vi "move X Relative.vi"(9 "Settings":T1, 10 "Speed X":i32, 11 "x mm":dbl) -> ()   [LabVIEW 2017]
uses:
  Settings/Settings-Control.ctl
  ICNC/ICNC2.lvlib
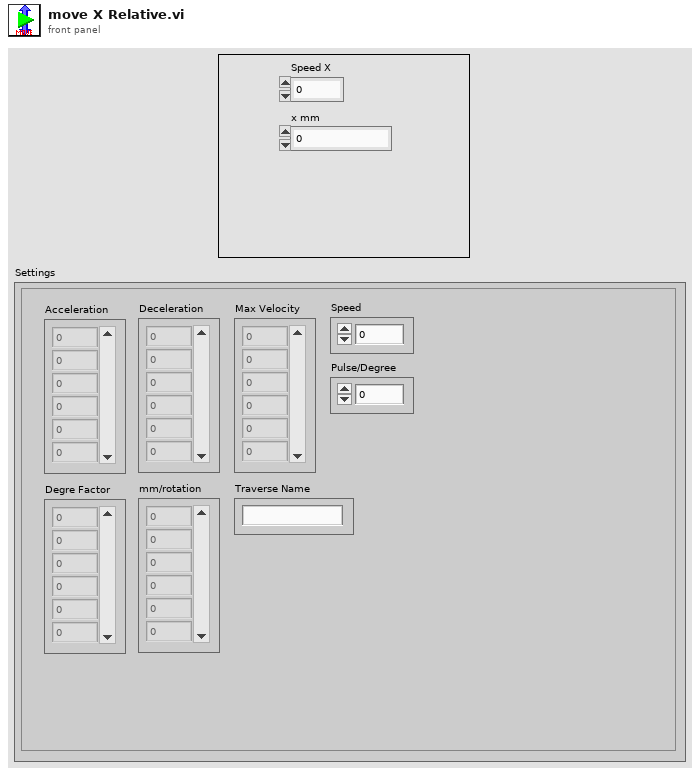
[diagram p1: front panel]
types:
  T1 = typedef "Settings-Control.ctl" = cluster{"Acceleration":dbl[], "Deceleration":dbl[], "Max Velocity":dbl[], "Speed":dbl, "Pulse/Degree":dbl, "Degre Factor":dbl[], "mm/rotation":dbl[], "Traverse Name":string}
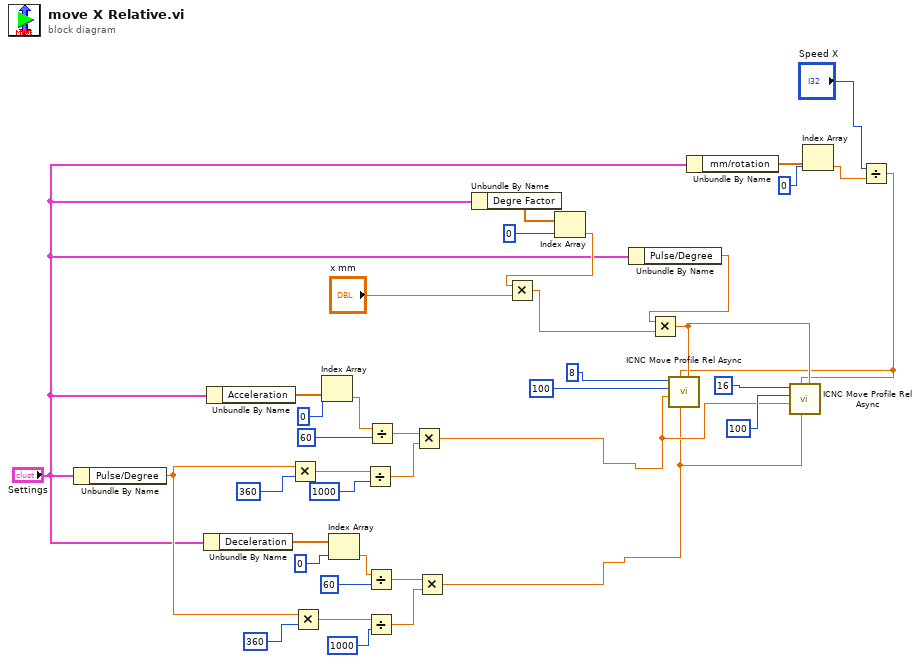
[diagram p0: block diagram]
diagram:
  n1 = Unbundle By Name("Settings") -> ("Pulse/Degree"=w20:dbl)
  n2 = Unbundle By Name("Settings") -> ("Deceleration"=w17:dbl[])
  n3 = Unbundle By Name("Settings") -> ("Acceleration"=w19:dbl[])
  n4 = Multiply(x=w20, y=360) -> (x*y=w28:dbl)
  n5 = Multiply(x=w20, y=360) -> (x*y=w27:dbl)
  n6 = Index Array(array=w19, index=0) -> (element=w11:dbl)
  n7 = Index Array(array=w17, index=0) -> (element=w10:dbl)
  n8 = Divide(x=w28, y=1000) -> (x/y=w38:dbl)
  n9 = Divide(x=w10, y=60) -> (x/y=w34:dbl)
  n10 = Divide(x=w27, y=1000) -> (x/y=w33:dbl)
  n11 = Divide(x=w11, y=60) -> (x/y=w29:dbl)
  n12 = Multiply(x=w29, y=w38) -> (x*y=w8:dbl)
  n13 = Multiply(x=w34, y=w33) -> (x*y=w7:dbl)
  n14 = Unbundle By Name("Settings") -> ("Degre Factor"=w12:dbl[])
  n15 = Index Array(array=w12, index=0) -> (element=w13:dbl)
  n16 = Multiply(x=w13, y="x mm") -> (x*y=w22:dbl)
  n17 = Unbundle By Name("Settings") -> ("Pulse/Degree"=w15:dbl)
  n18 = Multiply(x=w15, y=w22) -> (x*y=w21:dbl)
  n19 = Unbundle By Name("Settings") -> ("mm/rotation"=w6:dbl[])
  n20 = Index Array(array=w6, index=0) -> (element=w3:dbl)
  n21 = Divide(x="Speed X", y=w3) -> (x/y=w2:dbl)
  n22 = call <userlib>:"ICNC Move Profile Rel Async.vi"("Distance"=w21, "Decel"=w7, "Speed"=w2, "Accel"=w8, "FStartStop"=100, "Axe"=8) -> ()  [unwired: 4 in, 2 out]
  n23 = call <userlib>:"ICNC Move Profile Rel Async.vi"("Distance"=w21, "Decel"=w7, "Speed"=w2, "Accel"=w8, "FStartStop"=100, "Axe"=16) -> ()  [unwired: 4 in, 2 out]
